vi "WPI_SimpleGyro_Get Angle.vi"(8 "error in":errorcluster, 11 "SimpleGyroDevRef":T1) -> (0 "error out":errorcluster, 2 "Angle":dbl, 3 "SimpleGyroDevRef":T1)   [LabVIEW 2015, in "SimpleGyro.lvlib"]
doc: "Reads a sample from the SimpleGyro and makes it available to the rest of your program. Use this in your RobotMain.vi to provide WPI_RobotDriveHolonomicDrive.vi angle feedback."
uses:
  SimpleGyro.lvlib
  WPI_SimpleGyroDevRef.ctl
  <vilib>/Rock Robotics/SystemInterfaces/spilib/spi_bus.ctl
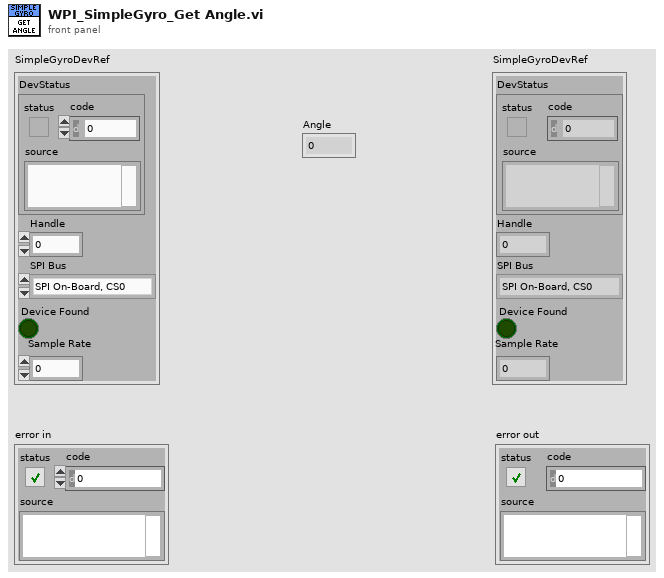
[diagram p1: front panel]
types:
  T1 = typedef "SimpleGyro.lvlib/WPI_SimpleGyroDevRef.ctl" = cluster{"DevStatus":errorcluster, "Handle":i32, "SPI Bus":T2, "Device Found":bool, "Sample Rate":dbl}
  T2 = typedef "spi_bus.ctl" = enum16{"SPI On-Board, CS0", "SPI On-Board, CS1", "SPI On-Board, CS2", "SPI On-Board, CS3", "SPI MXP", "Invalid"}
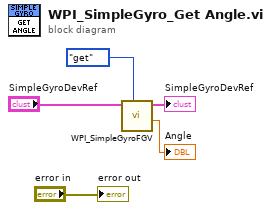
[diagram p0: block diagram]
diagram:
  n1 = call "WPI_SimpleGyroFGV.vi"("Operation"=enum16{"set", "get"}."get", "SimpleGyroDevRef"="SimpleGyroDevRef") -> ("Angle"=→"Angle":dbl, "SimpleGyroDevRef"=→"SimpleGyroDevRef":T1)  [unwired: 6 in, 2 out]
  "error out" <- "error in"
